vi "FTW-Example-SLASD-Core-Process.vi"() -> ()   [LabVIEW 2013, in "FTW-Example-SLASD-Core.lvclass"]
uses:
  FTW-Example-SLASD-Core.lvclass
  FTW-Example-SLASD-Core.lvclass/FTW-Example-SLASD-Core.ctl
  source/actor/Instance/FTW-ActorInstance.lvclass/FTW-ActorInstance.ctl
  <vilib>/nisyscfg/Close (System).vi
  <vilib>/nisyscfg/Close (Hardware).vi
  <vilib>/nisyscfg/Find Hardware.vi
  source/actor/JobSequencer/FTW-SEQ-Current.vi
  source/actor/Instance/FTW-ActorInstance.lvclass
  source/actor/Message/Request/FTW-Message-IncomingRequest.lvclass
  source/actor/Ether/FTW-Ether.lvclass
  <vilib>/nisyscfg/nisyscfg.lvlib
  <resource>/objmgr/nisysapi.rc
  <vilib>/NI_Real-Time Target Support.lvlib
  source/actor/Publisher/FTW-Publisher.lvclass
  Service/FTW-Example-Service.lvclass
panel:
  out "error out":errorcluster
  out "System Status":T1
  out "Elapsed Time":dbl format="%.6f sec"
  in  "Stop Button":bool
  # "avoid using Abort unless absolutely necessary"
  # "use this button to stop\nthe actor in RT dev mode\nsince user input events\ndo not work on RT"
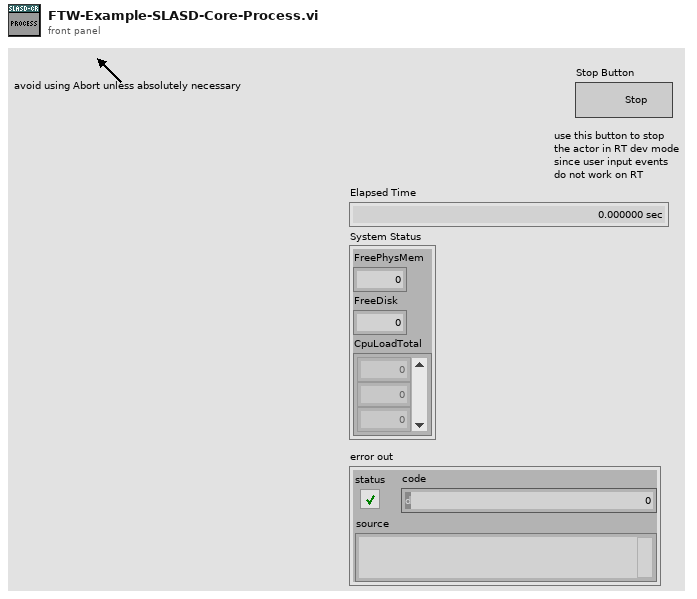
[diagram p1: front panel]
types:
  T1 = cluster{"FreePhysMem":dbl, "FreeDisk":dbl, "CpuLoadTotal":u32[]}
  T2 = cluster{"Incoming Requests":refnum<event-registration>, "Additional Registration Types":refnum<event-registration>}
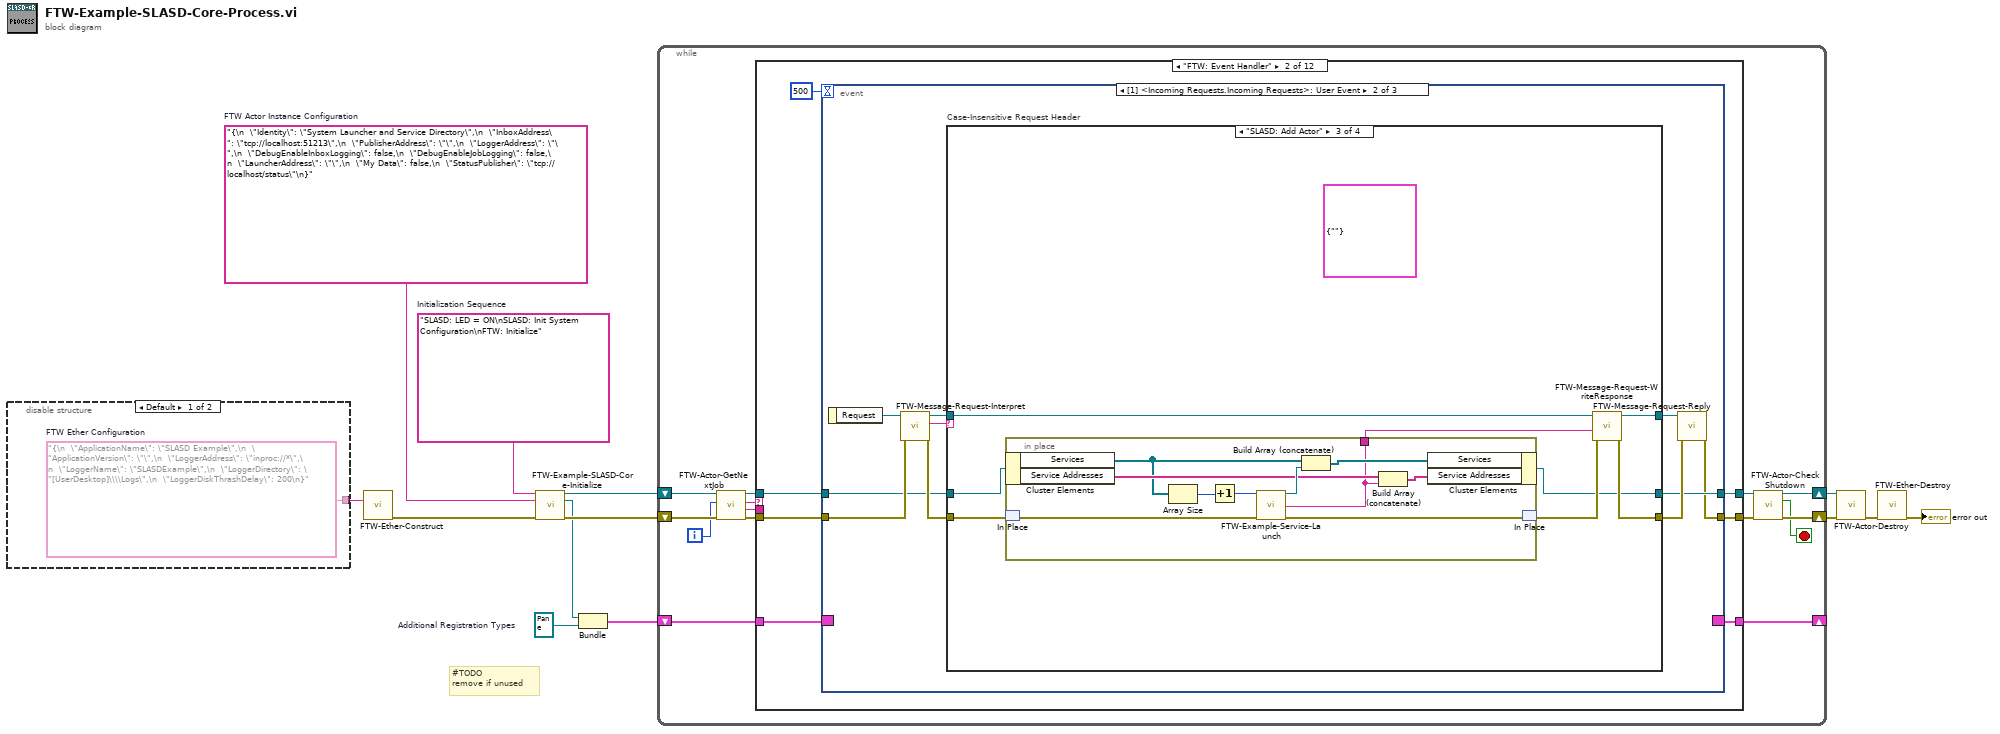
[diagram p0: block diagram]
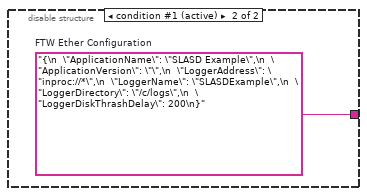
[diagram p2: hidden frame]
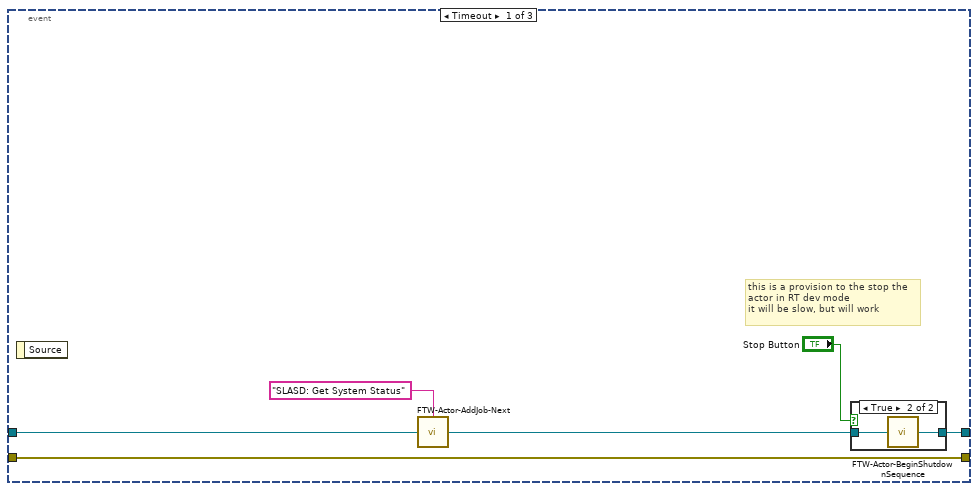
[diagram p4: hidden frame]
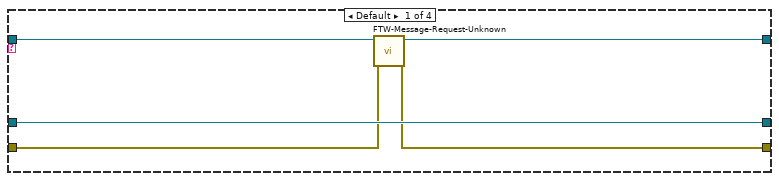
[diagram p6: hidden frame]
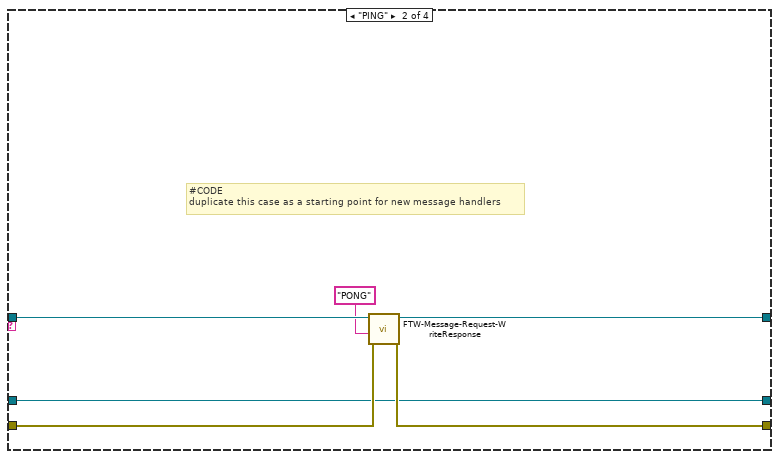
[diagram p7: hidden frame]
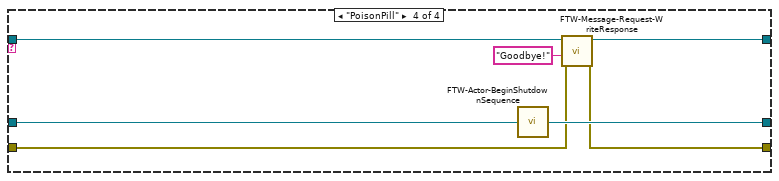
[diagram p8: hidden frame]
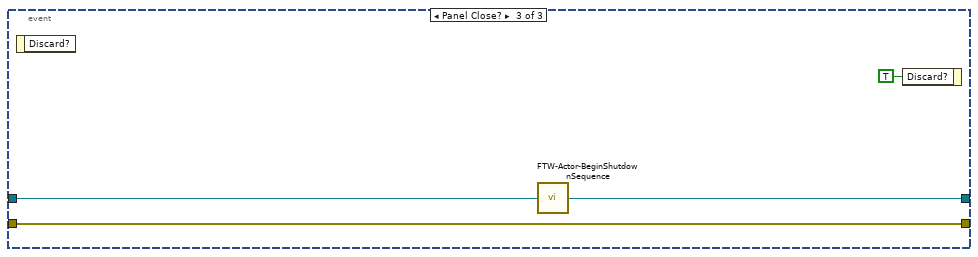
[diagram p9: hidden frame]
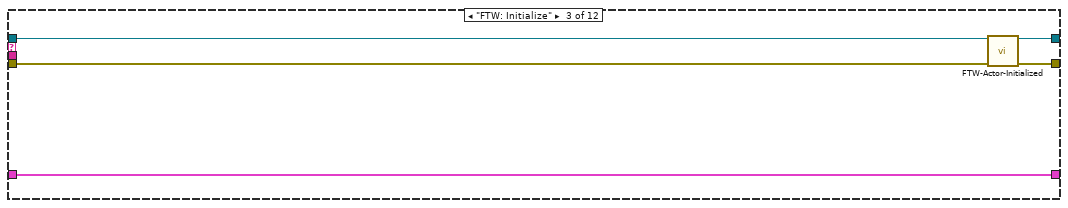
[diagram p10: hidden frame]
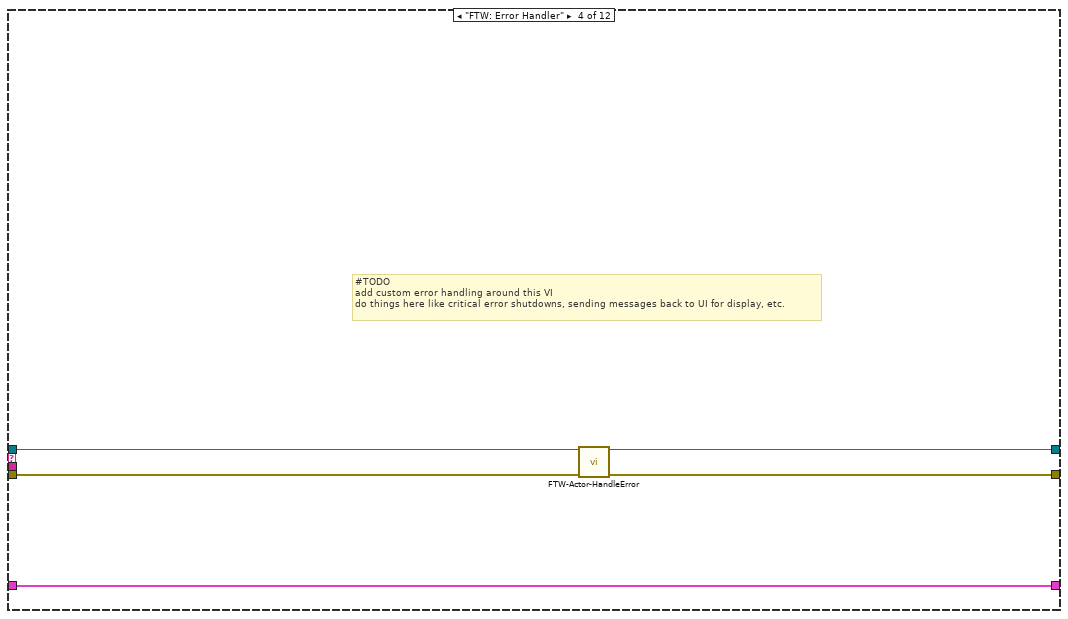
[diagram p11: hidden frame]
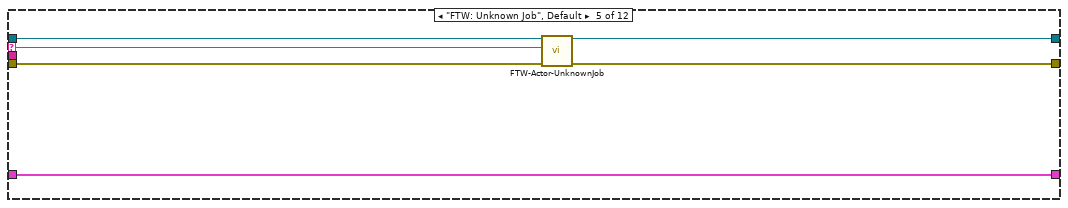
[diagram p12: hidden frame]
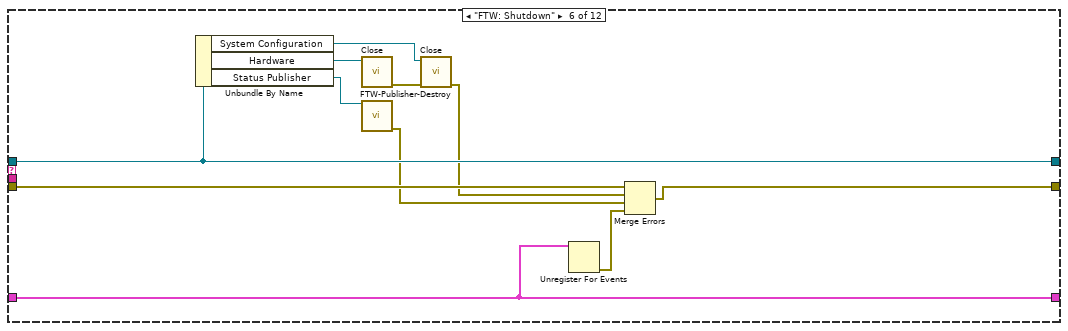
[diagram p13: hidden frame]
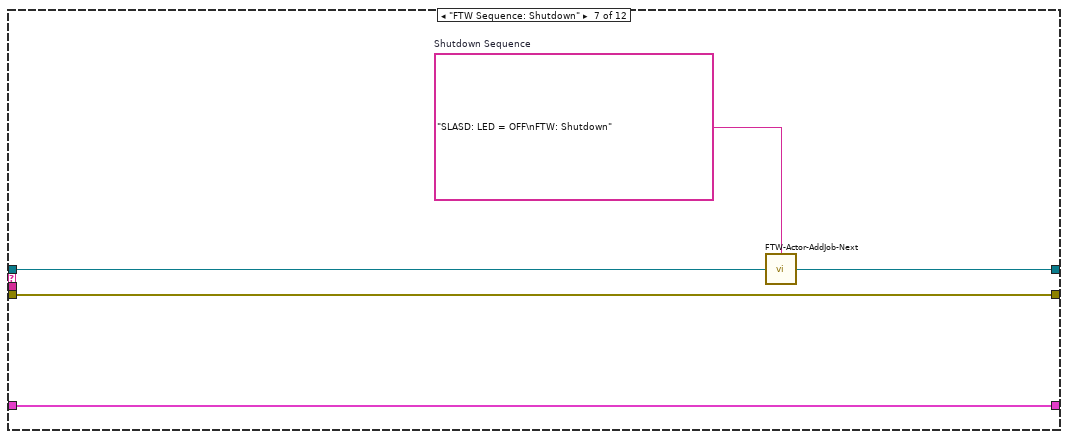
[diagram p14: hidden frame]
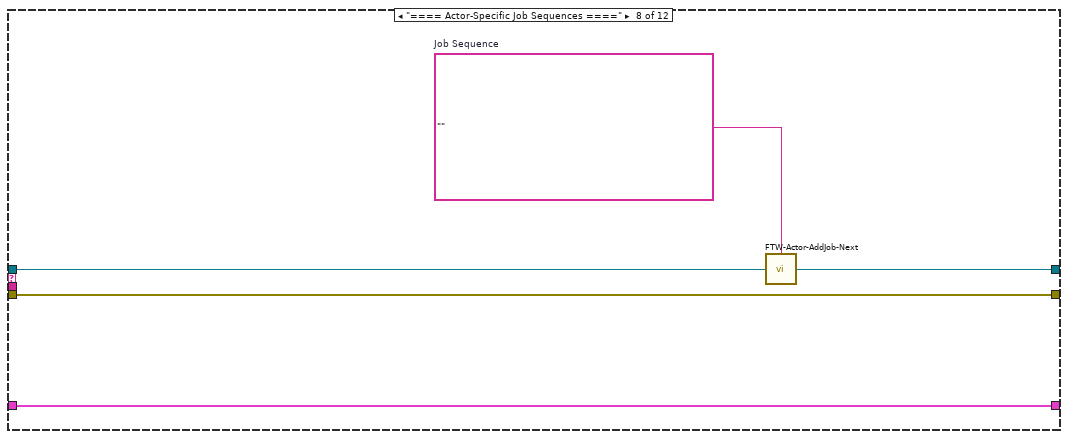
[diagram p15: hidden frame]
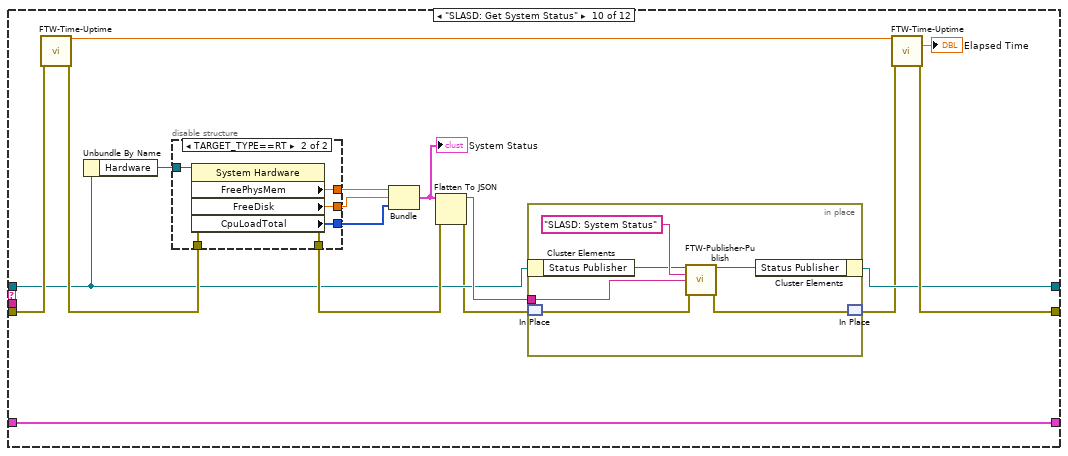
[diagram p17: hidden frame]
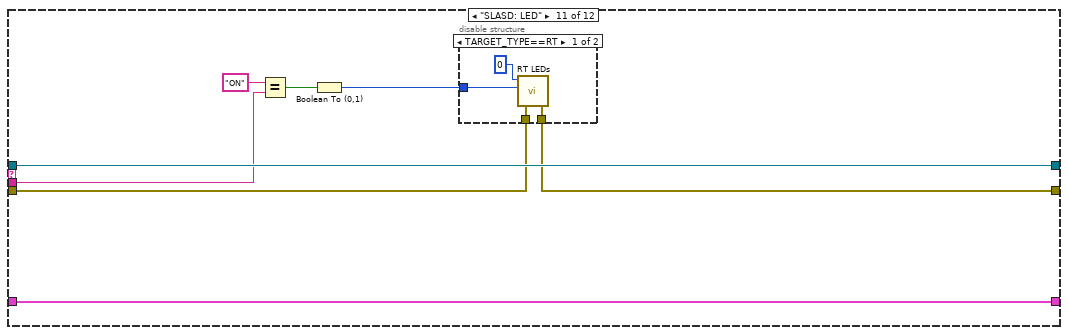
[diagram p19: hidden frame]
diagram:
  w5 = "{\n  \"Identity\": \"System Launcher and Service Directory\",\n  \"InboxAddress\": \"tcp://localhost:51213\",\n  \"PublisherAddress\": \"\",\n  \"LoggerAddress\": \"\",\n  \"DebugEnableInboxLogging\": false,\n  \"DebugEnableJobLogging\": false,\n  \"LauncherAddress\": \"\",\n  \"My Data\": false,\n  \"StatusPublisher\": \"tcp://localhost/status\"\n}"  # FTW Actor Instance Configuration
  w7 = refnum<event-registration> refnum  # Additional Registration Types
  w8 = "SLASD: LED = ON\nSLASD: Init System Configuration\nFTW: Initialize"  # Initialization Sequence
  # "#TODO\nremove if unused"
  n1 = disable-structure shown="Default" {
    disable-tunnel: [w14 w15] -> w2
    frame condition #0 {
      w14 = "{\n  \"ApplicationName\": \"SLASD Example\",\n  \"ApplicationVersion\": \"\",\n  \"LoggerAddress\": \"inproc://*\",\n  \"LoggerName\": \"SLASDExample\",\n  \"LoggerDirectory\": \"[UserDesktop]\\\\Logs\",\n  \"LoggerDiskThrashDelay\": 200\n}"  # FTW Ether Configuration
    }
    frame condition #1 (active) {
      w15 = "{\n  \"ApplicationName\": \"SLASD Example\",\n  \"ApplicationVersion\": \"\",\n  \"LoggerAddress\": \"inproc://*\",\n  \"LoggerName\": \"SLASDExample\",\n  \"LoggerDirectory\": \"/c/logs\",\n  \"LoggerDiskThrashDelay\": 200\n}"  # FTW Ether Configuration
    }
  }
  n2 = call "FTW-Ether-Construct.vi"("FTW Ether Configuration"=w2) -> ("error out"=w3:errorcluster)  [unwired: 14 in]
  n3 = call "FTW-Example-SLASD-Core-Initialize.vi"("Initialization Sequence"=w8, "FTW Actor Instance Configuration"=w5, "error in (no error)"=w3) -> ("Actor Template-Core out"=w13:refnum<class "FTW-Example-SLASD-Core.lvclass">, "Incoming Requests"=w4:refnum<event-registration>, "error out"=w9:errorcluster)  [unwired: 10 in]
  n4 = Bundle("Incoming Requests"=w4, "Additional Registration Types"=w7) -> (w6:T2)  [unwired: 1 in]
  n5 = while {
    shift-right: [w19] -> w11
    shift-left: w9 -> [w26]
    shift-right: [w16] -> _
    shift-left: w6 -> [w29]
    shift-right: [w21] -> w12
    shift-left: w13 -> [w28]
    i -> [w17]
    stop <- w18 stop-if-true
    n6 = call "FTW-Actor-GetNextJob.vi"("error in"=w26, "Jobs Performed"=w17, "FTW Actor Instance"=w28) -> ("error out"=w25:errorcluster, "Job Data"=w23:string, "Job Name"=w24:string, "FTW Actor Instance out"=w27:refnum<class "FTW-Example-SLASD-Core.lvclass">)  [unwired: 5 in]
    n7 = case shown="\"FTW: Event Handler\"" w24 {
      selector: w24 -> [_ _ _ _ w109 _ _ _ _ _ _ _]
      tunnel: [w31 w39 w99 w104 w112 w124 w129 w134 w138 w143 w169 w185] -> w20
      tunnel: w25 -> [w31 w38 w102 w106 w113 w125 w129 w134 w138 w144 w170 w186]
      tunnel: w29 -> [w32 w34 w103 w108 w114 w122 w130 w135 w137 w155 w176 w194]
      tunnel: [w32 w37 w103 w108 w114 w122 w130 w135 w137 w155 w176 w194] -> w16
      tunnel: w23 -> [_ _ _ _ _ _ _ _ _ _ w174 _]
      tunnel: [w30 w36 w100 w105 w110 w121 w127 w132 w136 w141 w175 w184] -> w22
      tunnel: w27 -> [w30 w35 w101 w107 w111 w121 w128 w133 w136 w142 w175 w193]
      frame "==== Featherweight Framework Jobs ====" {
      }
      frame "FTW: Event Handler" {
        n8 = event shown="[1] <Incoming Requests.Incoming Requests>: User Event" {
          selector: w34 -> [_ _ _]
          dyn-events: [_ _ _] -> w37
          timeout: 500 -> [_ _ _]
          tunnel: [w42 w51 w97] -> w39
          tunnel: w38 -> [w42 w50 w97]
          tunnel: [w45 w52 w95] -> w36
          tunnel: w35 -> [w43 w49 w96]
          event Timeout {
            # "this is a provision to the stop the\nactor in RT dev mode\nit will be slow, but will work"
            n9 = event-data() -> ()  [unwired: 1 in, 1 out]
            n10 = call "FTW-Actor-AddJob-Next.vi"("Add Next in Job Queue"="SLASD: Get System Status", "FTW Actor Instance"=w43) -> ("FTW Actor Instance out"=w41:refnum<class "FTW-Example-SLASD-Core.lvclass">)  [unwired: 2 in]
            n11 = case shown="True" "Stop Button" {
              tunnel: w41 -> [w46 w48]
              tunnel: [w46 w47] -> w45
              frame False {
              }
              frame True {
                n12 = call "FTW-Actor-BeginShutdownSequence.vi"("FTW Actor Instance"=w48) -> ("FTW Actor Instance out"=w47:refnum<class "FTW-Example-SLASD-Core.lvclass">)  [unwired: 3 in]
              }
            }
          }
          event User Event {
            n13 = event-data() -> ("Request"=w53:refnum<class "FTW-Message-IncomingRequest.lvclass">)  [unwired: 1 in]
            n14 = call "FTW-Message-Request-Interpret.vi"("error in"=w50, "FTW Incoming Request"=w53) -> ("error out"=w58:errorcluster, "Request Header"=w56:string, "FTW Incoming Request out"=w55:refnum<class "FTW-Message-IncomingRequest.lvclass">)  [unwired: 5 in, 2 out]
            n15 = case "Case-Insensitive Request Header" shown="\"SLASD: Add Actor\"" w56 {
              tunnel: [w61 w67 w76 w91] -> w57
              tunnel: w58 -> [w62 w68 w74 w93]
              tunnel: [w63 w66 w71 w94] -> w52
              tunnel: w49 -> [w63 w66 w72 w92]
              tunnel: w55 -> [w60 w69 w77 w90]
              tunnel: [w59 w65 w75 w89] -> w54
              frame Default {
                n16 = call "FTW-Message-Request-Unknown.vi"("error in"=w62, "FTW Incoming Request"=w60) -> ("error out"=w61:errorcluster, "FTW Incoming Request Out"=w59:refnum<class "FTW-Message-IncomingRequest.lvclass">)  [unwired: 8 in]
              }
              frame "PING" {
                # "#CODE\nduplicate this case as a starting point for new message handlers"
                n17 = call "FTW-Message-Request-WriteResponse.vi"("error in"=w68, "Response Body"="PONG" ("Response Header"), "FTW Incoming Request"=w69) -> ("error out"=w67:errorcluster, "FTW Incoming Request out"=w65:refnum<class "FTW-Message-IncomingRequest.lvclass">)  [unwired: 7 in]
              }
              frame "SLASD: Add Actor" {
                (unwired) cluster{string} {""}
                n18 = in-place {
                  in-place-border: [w78] -> w70
                  n19 = in-place-cluster #1(w72) -> ("Services"=w81:refnum<class "FTW-Example-Service.lvclass">[], "Service Addresses"=w82:string[])
                  n20 = in-place-match #2(w74) -> (w87:errorcluster)
                  n21 = Array Size(array=w81) -> (size(s)=w80:i32)
                  n22 = Increment(x=w80) -> (x+1=w79:i32)
                  n23 = call "FTW-Example-Service-Launch.vi"("Number"=w79, "error in"=w87) -> ("FTW Actor Connector"=w85:refnum<class "FTW-Example-Service.lvclass">, "Instance Inbox Address"=w78:string, "error out"=w86:errorcluster)  [unwired: 10 in, 1 out]
                  n24 = Build Array (concatenate)(w81, w85) -> (w84:refnum<class "FTW-Example-Service.lvclass">[])
                  n25 = Build Array (concatenate)(w82, w78) -> (w83:string[])
                  n26 = in-place-cluster #1("Services"=w84, "Service Addresses"=w83) -> (w71:refnum<class "FTW-Example-SLASD-Core.lvclass">)
                  n27 = in-place-match #2(w86) -> (w73:errorcluster)
                }
                n28 = call "FTW-Message-Request-WriteResponse.vi"("error in"=w73, "Response Body"=w70, "FTW Incoming Request"=w77) -> ("error out"=w76:errorcluster, "FTW Incoming Request out"=w75:refnum<class "FTW-Message-IncomingRequest.lvclass">)  [unwired: 7 in]
              }
              frame "PoisonPill" {
                n29 = call "FTW-Actor-BeginShutdownSequence.vi"("FTW Actor Instance"=w92) -> ("FTW Actor Instance out"=w94:refnum<class "FTW-Example-SLASD-Core.lvclass">)  [unwired: 3 in]
                n30 = call "FTW-Message-Request-WriteResponse.vi"("error in"=w93, "Response Body"="Goodbye!", "FTW Incoming Request"=w90) -> ("error out"=w91:errorcluster, "FTW Incoming Request out"=w89:refnum<class "FTW-Message-IncomingRequest.lvclass">)  [unwired: 7 in]
              }
            }
            n31 = call "FTW-Message-Request-Reply.vi"("FTW: Reply Error"=w57, "FTW Incoming Request"=w54) -> ("error out"=w51:errorcluster)  [unwired: 8 in, 1 out]
          }
          event Panel Close? {
            n32 = event-data() -> ()  [unwired: 1 in, 1 out]
            n33 = call "FTW-Actor-BeginShutdownSequence.vi"("FTW Actor Instance"=w96) -> ("FTW Actor Instance out"=w95:refnum<class "FTW-Example-SLASD-Core.lvclass">)  [unwired: 3 in]
            n34 = event-data("Discard?"=TRUE) -> ()  [unwired: 1 in, 1 out]
          }
        }
      }
      frame "FTW: Initialize" {
        n35 = call-dynamic "FTW-Actor-Initialized.vi"("FTW Actor Instance"=w101, "error in"=w102) -> ("FTW Actor Instance out"=w100:refnum<class "FTW-Example-SLASD-Core.lvclass">, "error out"=w99:errorcluster)  [unwired: 12 in]
      }
      frame "FTW: Error Handler" {
        # "#TODO\nadd custom error handling around this VI\ndo things here like critical error shutdowns, sending messages back to UI for display, etc."
        n36 = call-dynamic "FTW-Actor-HandleError.vi"("FTW Actor Instance"=w107, "error in"=w106) -> ("FTW Actor Instance out"=w105:refnum<class "FTW-Example-SLASD-Core.lvclass">, "error out"=w104:errorcluster)  [unwired: 10 in, 2 out]
      }
      frame "FTW: Unknown Job", Default {
        n37 = call-dynamic "FTW-Actor-UnknownJob.vi"("FTW Actor Instance"=w111, "Unknown Job"=w109, "error in"=w113) -> ("FTW Actor Instance out"=w110:refnum<class "FTW-Example-SLASD-Core.lvclass">, "error out"=w112:errorcluster)  [unwired: 11 in]
      }
      frame "FTW: Shutdown" {
        n38 = Unbundle By Name(w121) -> ("System Configuration"=w118:refnum<k21>, "Hardware"=w120:refnum<k20>, "Status Publisher"=w116:refnum<class "FTW-Publisher.lvclass">)
        n39 = call-poly <vilib>:"Close.vi"("resource in"=w120) -> ("error out"=w119:errorcluster)  [unwired: 10 in]
        n40 = call "FTW-Publisher-Destroy.vi"("FTW-Publisher In"=w116) -> ("error out"=w115:errorcluster)  [unwired: 14 in]
        n41 = call-poly <vilib>:"Close.vi"("error in (no error)"=w119, "session in"=w118) -> ("error out"=w117:errorcluster)  [unwired: 9 in]
        n42 = Unregister For Events(event registration refnum=w122) -> (error out=w123:errorcluster)  [unwired: 1 in]
        n43 = Merge Errors(w125, w117, w115, w123) -> (w124:errorcluster)
      }
      frame "FTW Sequence: Shutdown" {
        w126 = "SLASD: LED = OFF\nFTW: Shutdown"  # Shutdown Sequence
        n44 = call "FTW-Actor-AddJob-Next.vi"("Add Next in Job Queue"=w126, "FTW Actor Instance"=w128) -> ("FTW Actor Instance out"=w127:refnum<class "FTW-Example-SLASD-Core.lvclass">)  [unwired: 2 in]
      }
      frame "==== Actor-Specific Job Sequences ====" {
        w131 = ""  # Job Sequence
        n45 = call "FTW-Actor-AddJob-Next.vi"("Add Next in Job Queue"=w131, "FTW Actor Instance"=w133) -> ("FTW Actor Instance out"=w132:refnum<class "FTW-Example-SLASD-Core.lvclass">)  [unwired: 2 in]
      }
      frame "==== Actor-Specific Jobs ====" {
      }
      frame "SLASD: Get System Status" {
        n46 = call "FTW-Time-Uptime.vi"("error in"=w144) -> ("Current Uptime"=w146:dbl, "error out"=w147:errorcluster)  [unwired: 12 in, 1 out]
        n47 = Unbundle By Name(w142) -> ("Hardware"=w154:refnum<k20>)
        n48 = disable-structure shown="TARGET_TYPE==RT" {
          disable-tunnel: w147 -> [w162 w168]
          disable-tunnel: [_ w167] -> w151
          disable-tunnel: w154 -> [_ w166]
          disable-tunnel: [_ w165] -> w152
          disable-tunnel: [_ w164] -> w153
          disable-tunnel: [w162 w163] -> w150
          frame condition #0 {
          }
          frame condition #1 (active) {
            n49 = property class="System Hardware"(reference=w166, error in=w168) -> (error out=w163:errorcluster, "FreePhysMem"=w164:dbl, "FreeDisk"=w165:dbl, "CpuLoadTotal"=w167:u32[])  [unwired: 1 out]
          }
        }
        n50 = Bundle("FreePhysMem"=w153, "FreeDisk"=w152, "CpuLoadTotal"=w151) -> (w149:T1)  [unwired: 1 in]
        "System Status" <- w149
        n51 = Flatten To JSON(anything=w149, error in (no error)=w150) -> (JSON string=w148:string, 11:w140:errorcluster)  [unwired: 1 in]
        n52 = in-place {
          in-place-border: w148 -> [w161]
          n53 = in-place-cluster #3(w142) -> ("Status Publisher"=w159:refnum<class "FTW-Publisher.lvclass">)
          n54 = in-place-match #4(w140) -> (w157:errorcluster)
          n55 = call "FTW-Publisher-Publish.vi"("FTW-Publisher In"=w159, "Header"="SLASD: System Status" ("Message Header"), "Body"=w161, "error in"=w157) -> ("FTW-Publisher Out"=w158:refnum<class "FTW-Publisher.lvclass">, "error out"=w156:errorcluster)  [unwired: 10 in]
          n56 = in-place-cluster #3("Status Publisher"=w158) -> (w141:refnum<class "FTW-Example-SLASD-Core.lvclass">)
          n57 = in-place-match #4(w156) -> (w139:errorcluster)
        }
        n58 = call "FTW-Time-Uptime.vi"("Previous Uptime"=w146, "error in"=w139) -> ("Elapsed Time"=→"Elapsed Time":dbl, "error out"=w143:errorcluster)  [unwired: 11 in, 1 out]
      }
      frame "SLASD: LED" {
        n59 = Equal?(x="ON", y=w174) -> (x = y?=w172:bool)
        n60 = Boolean To (0,1)(Boolean=w172) -> (0, 1=w171:i16)
        n61 = disable-structure shown="TARGET_TYPE==RT" {
          disable-tunnel: w171 -> [w179 _]
          disable-tunnel: w170 -> [w178 w181]
          disable-tunnel: [w177 w181] -> w169
          frame condition #0 (active) {
            n62 = call <vilib>:"RT LEDs.vi"("error in (no error)"=w178, "State"=w179, "LED Num"=0) -> ("error out"=w177:errorcluster)  [unwired: 3 in, 1 out]
          }
          frame condition #1 {
          }
        }
      }
      frame "SLASD: Init System Configuration" {
        # "close unused references"
        n63 = call <vilib>:"Initialize Session.vi"("error in (no error)"=w186) -> ("error out"=w192:errorcluster, "session out"=w191:refnum<k21>)  [unwired: 9 in]
        n64 = call-poly <vilib>:"Find.vi"("error in (no error)"=w192, "session in"=w191) -> ("error out"=w188:errorcluster, "resources out"=w190:refnum<k20>[], "session out"=w183:refnum<k21>)  [unwired: 6 in, 1 out]
        n65 = Delete From Array(array=w190, index=0) -> (deleted portion=w182:refnum<k20>, array with subset deleted=w187:refnum<k20>[])  [unwired: 1 in]
        n66 = for {
          tunnel: w187 -> [w197] mode=indexing
          shift-right: [w195] -> w185
          shift-left: w188 -> [w196]
          n67 = call-poly <vilib>:"Close.vi"("error in (no error)"=w196, "resource in"=w197) -> ("error out"=w195:errorcluster)  [unwired: 9 in]
        }
        n68 = Bundle By Name(cluster=w193, "System Configuration"=w183, "Hardware"=w182) -> (w184:refnum<class "FTW-Example-SLASD-Core.lvclass">)
      }
    }
    n69 = call "FTW-Actor-CheckShutdown.vi"("FTW Actor Instance"=w22, "error in"=w20) -> ("FTW Actor Instance out"=w21:refnum<class "FTW-Example-SLASD-Core.lvclass">, "Shutdown?"=w18:bool, "error out"=w19:errorcluster)  [unwired: 11 in]
  }
  n70 = call-dynamic "FTW-Actor-Destroy.vi"("FTW Actor Instance"=w12, "error in"=w11) -> ("error out"=w10:errorcluster)  [unwired: 13 in]
  n71 = call "FTW-Ether-Destroy.vi"("error in"=w10) -> ("error out"=→"error out":errorcluster)  [unwired: 14 in]
